vi "Kalman_Filter_Setter_Offline.vi"(8 "error in (no error)":errorcluster, 10 "Filter Constants":T1, 11 "Kalman_Filter in":refnum<class "Kalman_Filter.lvclass">) -> (0 "error out":errorcluster, 3 "Kalman_Filter out":refnum<class "Kalman_Filter.lvclass">)   [LabVIEW 2021, in "Kalman_Filter.lvclass"]
uses:
  Kalman_Filter.lvclass
  Kalman_Filter.lvclass/Kalman_Filter.ctl
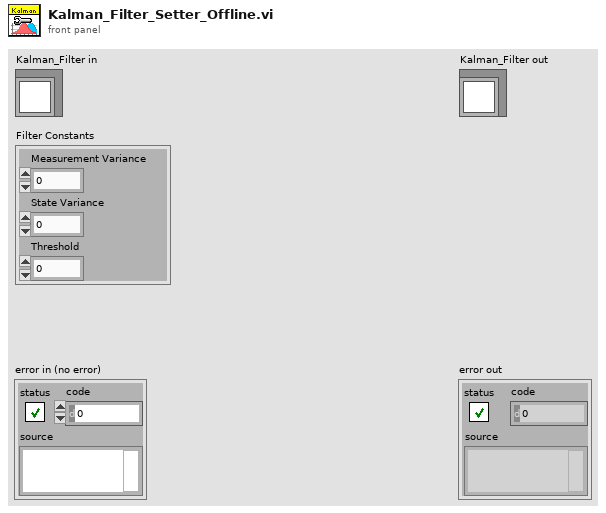
[diagram p1: front panel]
types:
  T1 = cluster{"Measurement Variance":dbl, "State Variance":dbl, "Threshold":dbl}
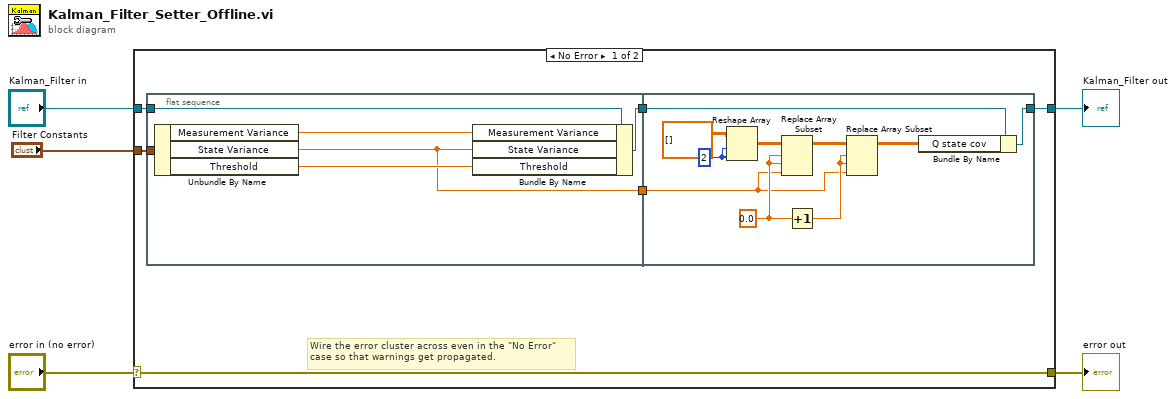
[diagram p0: block diagram]
diagram:
  n1 = case shown="No Error" "error in (no error)" {
    selector: "error in (no error)" -> [w11 w29]
    tunnel: [w11 w29] -> w4
    tunnel: [w9 w28] -> w2
    tunnel: "Kalman_Filter in" -> [w10 w28]
    tunnel: "Filter Constants" -> [w8 _]
    frame No Error {
      # "Wire the error cluster across even in the \"No Error\"\ncase so that warnings get propagated."
      n2 = flat-sequence {
        tunnel: w10 -> [w17]
        tunnel: w8 -> [w15]
        tunnel: [w16] -> w7
        tunnel: [w12] -> w6
        tunnel: [w19] -> w9
        tunnel: w7 -> [w21]
        tunnel: w6 -> [w22]
        frame #0 {
          n3 = Unbundle By Name(w15) -> ("Measurement Variance"=w14:dbl, "State Variance"=w12:dbl, "Threshold"=w13:dbl)
          n4 = Bundle By Name(cluster=w17, "Measurement Variance"=w14, "State Variance"=w12, "Threshold"=w13) -> (w16:refnum<class "Kalman_Filter.lvclass">)
        }
        frame #1 {
          w24 = 0.0 ("State Variance")
          w18 = 2 ("dimension size")
          n5 = Reshape Array(dbl[][] [], w18, w18) -> (w26:dbl[][])
          n6 = Replace Array Subset(array=w26, new element=w22, index (row)=w24, index (col)=w24) -> (w25:dbl[][])
          n7 = Increment(x=w24) -> (x+1=w23:dbl)
          n8 = Replace Array Subset(array=w25, new element=w22, index (row)=w23, index (col)=w23) -> (w20:dbl[][])
          n9 = Bundle By Name(cluster=w21, "Q state cov"=w20) -> (w19:refnum<class "Kalman_Filter.lvclass">)
        }
      }
    }
    frame Error {
    }
  }
  "error out" <- w4
  "Kalman_Filter out" <- w2
